vi "for.vi"() -> ()   [LabVIEW 2020]
panel:
  out "Thermometer":dbl(slide) scale=0.0..100.0
  out "Iteraciones":i32
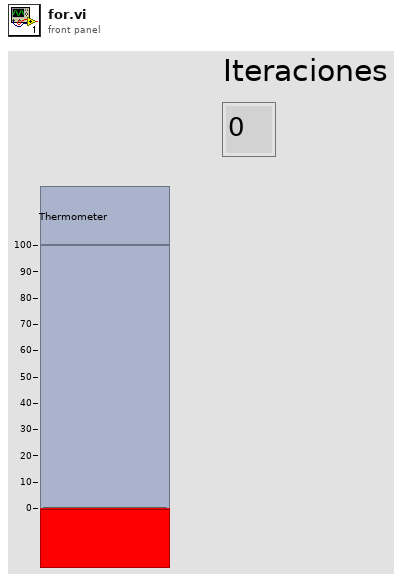
[diagram p1: front panel]
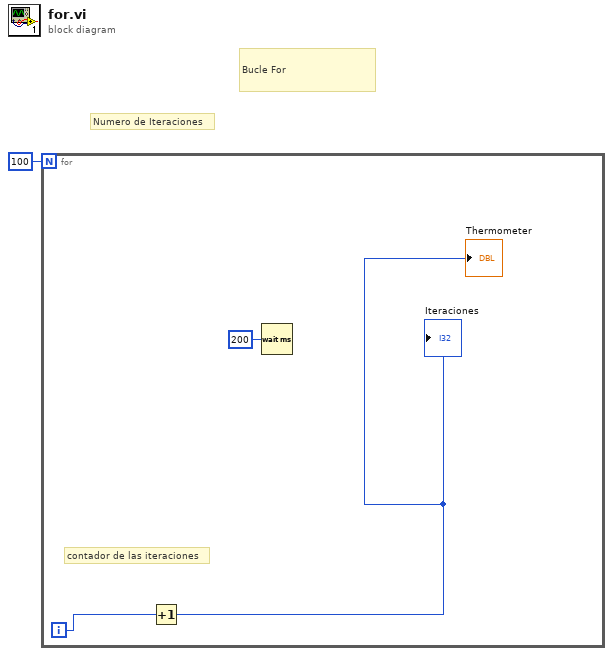
[diagram p0: block diagram]
diagram:
  # "Bucle For"
  # "Numero de Iteraciones"
  n1 = for {
    N: 100 -> [_]
    i -> [w3]
    # "contador de las iteraciones"
    n2 = Increment(x=w3) -> (x+1=→"Iteraciones" →"Thermometer":i32)
    n3 = Wait (ms)(milliseconds to wait=u32 200) -> ()  [unwired: 1 out]
  }
